vi "Open Hardware.vi"(8 "error in (no error)":errorcluster, 11 "Inst.MOTOR in":refnum<class "Inst.MOTOR.lvclass">) -> (0 "error out":errorcluster, 3 "Inst.MOTOR out":refnum<class "Inst.MOTOR.lvclass">)   [LabVIEW 2019, in "Inst.MOTOR.lvclass"]
uses:
  Inst.MOTOR.lvclass
  Inst.MOTOR.lvclass/Inst.MOTOR.ctl
  <vilib>/Instr/_visa.llb/VISA Configure Serial Port (Instr).vi
  <userlib>/LevyLab/Instrument Framework/Instrument Types/VSource/Instrument.VSource.lvclass
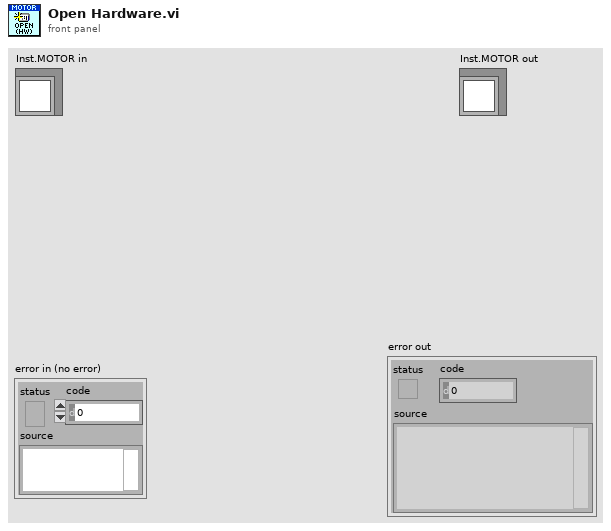
[diagram p1: front panel]
types:
  T1 = typedef "Serial - ASCII Characters.ctl" = enum16{"NUL", "SOH", "STX", "ETX", "EOT", "ENQ", "ACK", "BEL", "BS", "HT", "LF", "VT", "FF", "CR", "SO", "SI", "DLE", "DC1", "DC2", "DC3", "DC4", "NAK", "SYN", "ETB", "CAN", "EM", "SUB", "ESC", "FS", "GS", "RS", "US", "SP", "!", "\"", "#", "$", "%", "&", "'", "(", ")", "*", "+", ",", "- (-)", ".", "/", "0", "1", "2", "3", "4", "5", "6", "7", "8", "9", ":", ";", "<", "=", ">", "?", "@", "A", "B", "C", "D", "E", "F", "G", "H", "I", "J", "K", "L", "M", "N", "O", "P", "Q", "R", "S", "T", "U", "V", "W", "X", "Y", "Z", "[", "\\", "]", "^", "_", "`", "a", "b", "c", "d", "e", "f", "g", "h", "i", "j", "k", "l", "m", "n", "o", "p", "q", "r", "s", "t", "u", "v", "w", "x", "y", "z", "{", "|", "}", "~"}
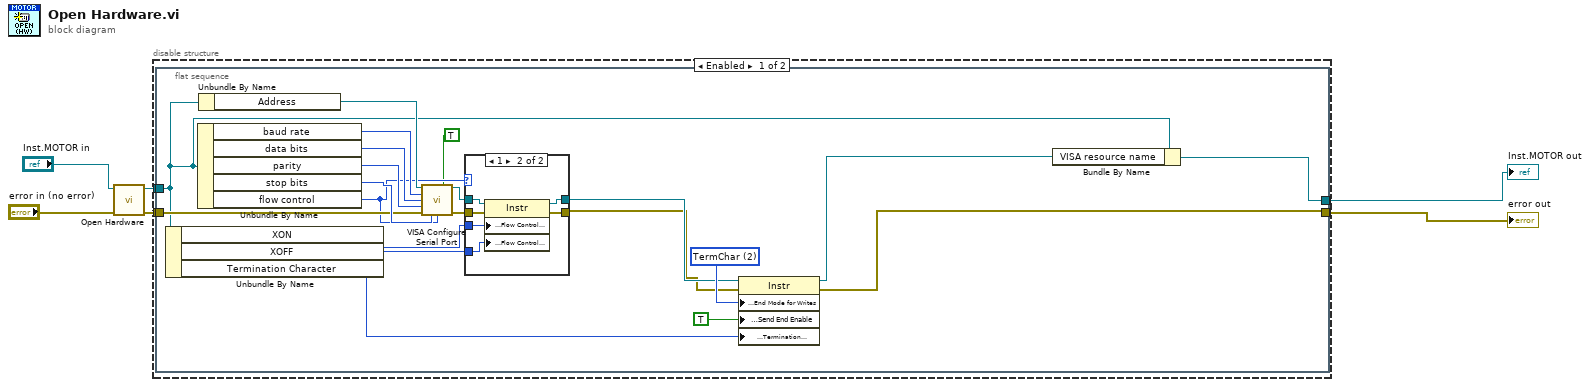
[diagram p0: block diagram]
diagram:
  n1 = call-parent "Open Hardware.vi"("error in (no error)"="error in (no error)", "Instrument in"="Inst.MOTOR in") -> ("error out"=w2:errorcluster, "Instrument out"=w4:refnum<class "Inst.MOTOR.lvclass">)  [unwired: 8 in]
  n2 = disable-structure shown="Enabled" {
    disable-tunnel: w4 -> [w10 w41]
    disable-tunnel: [w9 w40] -> w3
    disable-tunnel: w2 -> [w8 w40]
    disable-tunnel: [w7 w41] -> w1
    frame Enabled {
      n3 = flat-sequence {
        tunnel: w10 -> [w19]
        tunnel: [w13] -> w9
        tunnel: w8 -> [w26]
        tunnel: [w20] -> w7
        frame #0 {
          w17 = u16 2 items=["None", "LastBit", "TermChar", "Break"] ("Serial Settings:Serial End Mode for Writes")
          n4 = Unbundle By Name(w19) -> ("XON"=w22:T1, "XOFF"=w23:T1, "Termination Character"=w16:u8)
          n5 = Unbundle By Name(w19) -> ("baud rate"=w31:u32, "data bits"=w30:u16, "parity"=w29:enum16{"None", "Odd", "Even", "Mark", "Space"}, "stop bits"=w28:u16, "flow control"=w21:u16)
          n6 = Unbundle By Name(w19) -> ("Address"=w27:refnum<visa-resource-name>)
          n7 = call-poly "VISA Configure Serial Port"("VISA resource name"=w27, "Enable Termination\nChar (T)"=TRUE ("Enable Termination\nChar (T)"), "baud rate (9600)"=w31, "data bits (8)"=w30, "parity (0:none)"=w29, "error in (no error)"=w26, "stop bits (10: 1 bit)"=w28, "flow control (0:none)"=w21) -> ("VISA resource name out"=w24:refnum<visa-resource-name>, "error out"=w25:errorcluster)  [unwired: 2 in, 4 out]
          n8 = case shown="1" w21 {
            tunnel: [w32 w39] -> w14
            tunnel: [w33 w38] -> w15
            tunnel: w25 -> [w32 w37]
            tunnel: w24 -> [w33 w36]
            tunnel: w22 -> [_ w35]
            tunnel: w23 -> [_ w34]
            frame Default {
            }
            frame 1 {
              n9 = property class="Instr"(reference=w36, error in=w37, "Serial Settings:Flow Control XON Character"=w35, "Serial Settings:Flow Control XOFF Character"=w34) -> (reference out=w38:refnum<visa-resource-name>, error out=w39:errorcluster)
            }
          }
          n10 = property class="Instr"(reference=w15, error in=w14, "Serial Settings:End Mode for Writes"=w17, "Message Based Settings:Send End Enable"=TRUE, "Message Based Settings:Termination Character"=w16) -> (reference out=w12:refnum<visa-resource-name>, error out=w13:errorcluster)
          n11 = Bundle By Name(cluster=w19, "VISA resource name"=w12) -> (w20:refnum<class "Inst.MOTOR.lvclass">)
        }
      }
    }
    frame Disabled {
    }
  }
  "error out" <- w3
  "Inst.MOTOR out" <- w1
